vi "_r_n.vi"() -> (2 "command":string)   [LabVIEW 2023]
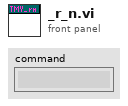
[diagram p1: front panel]
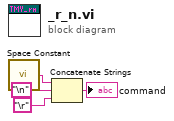
[diagram p0: block diagram]
diagram:
  n1 = call <vilib>:"Space Constant.vi"() -> ("String"=w2:string)
  n2 = Concatenate Strings(w2, "\n", "\r") -> (→"command":string)
